vi "Serial_Read (2).vi"() -> ()   [LabVIEW 2010]
uses:
  <vilib>/Instr/_visa.llb/VISA Configure Serial Port (Instr).vi
  <vilib>/Analysis/NI_AALPro.lvlib
panel:
  in  "Tab Control":T1(tab)
  in  "Serial Input":refnum<visa-resource-name>="COM4"
  in  "data bits":u16=8 min=5 max=8 step=1
  in  "parity":u16(ring) items=["None", "Odd", "Even", "Mark", "Space"]
  in  "stop bits":u16(ring)=10 items=["1.0"=10, "1.5"=15, "2.0"=20]
  in  "flow control":u16(ring) items=["None"=0, "XON/XOFF"=1, "RTS/CTS"=2, "DTR/DSR"=4]
  in  "delay before read (ms)":u32=500
  in  "byte count":u32=500
  out "Incoming Serial String":string
  out "Time":string
  out "Date":string
  in  "stop":bool
  out "return count":u32
  in  "baud rate (9600)":u32=9600
  out "N2O is FLAT":bool
  out "Rolling CO Slope Fit":cluster{i32[], "Best Linear Fit":dbl[]}[](graph)
  out "CO":dbl(graph)=0.310407
  out "N2O":dbl(graph)
  out "H2O":dbl(graph)
  out "CO PPM":string
  out "N2O PPM":string
  out "H2O PPM":string
  out "CO DRY":dbl(graph)
  out "CO DRY":string
  out "N2O DRY 2":string
  out "N2O DRY":dbl(graph)
  in  "Average Points":i32
  out "slope":dbl
  out "Rolling N2O Slope Fit 2":cluster{i32[], "Best Linear Fit":dbl[]}[](graph)
  out "slope 2":dbl
  in  "N2O Low Limit":dbl
  in  "CO High Limit":dbl
  out "CO is FLAT":bool
  in  "CO Low Limit":dbl
  in  "N2O High Limit":dbl
  out "CELL TEMP":string
  out "CELL TEMPERATURE":dbl(graph)
  out "AMBIENT TEMPERATURE":dbl(graph)
  out "AMBIENT TEMP":string
  out "AIN5":dbl(graph)
  out "SUPERCOOL TEMP":string
  out "LINE LOCK":dbl(graph)
  out "LINELOCK - LASER CONTROL VOLTAGE":string
  out "PRESSURE":dbl(graph)
  out "PRESSURE 2":string
  out "SuperCool Temperature":dbl
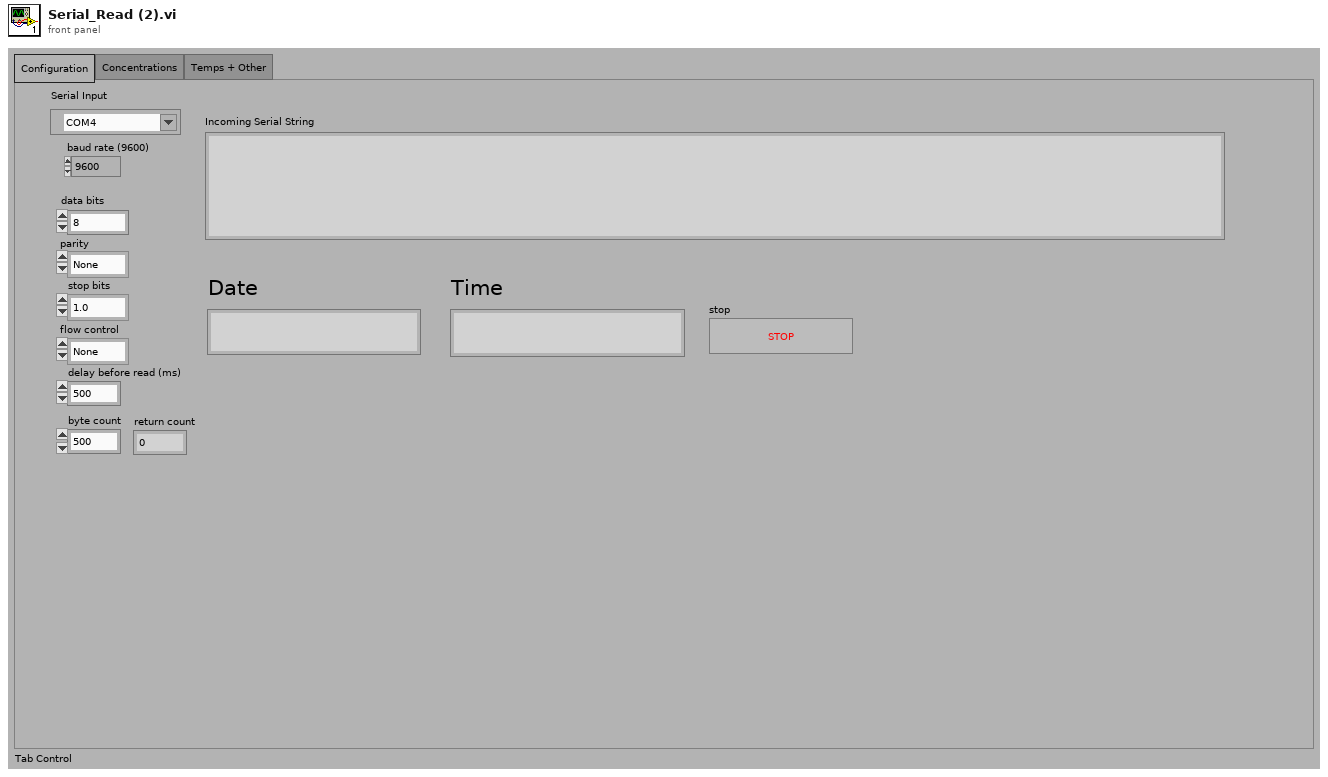
[diagram p1: front panel]
types:
  T1 = enum32{"Configuration", "Concentrations", "Temps + Other"}
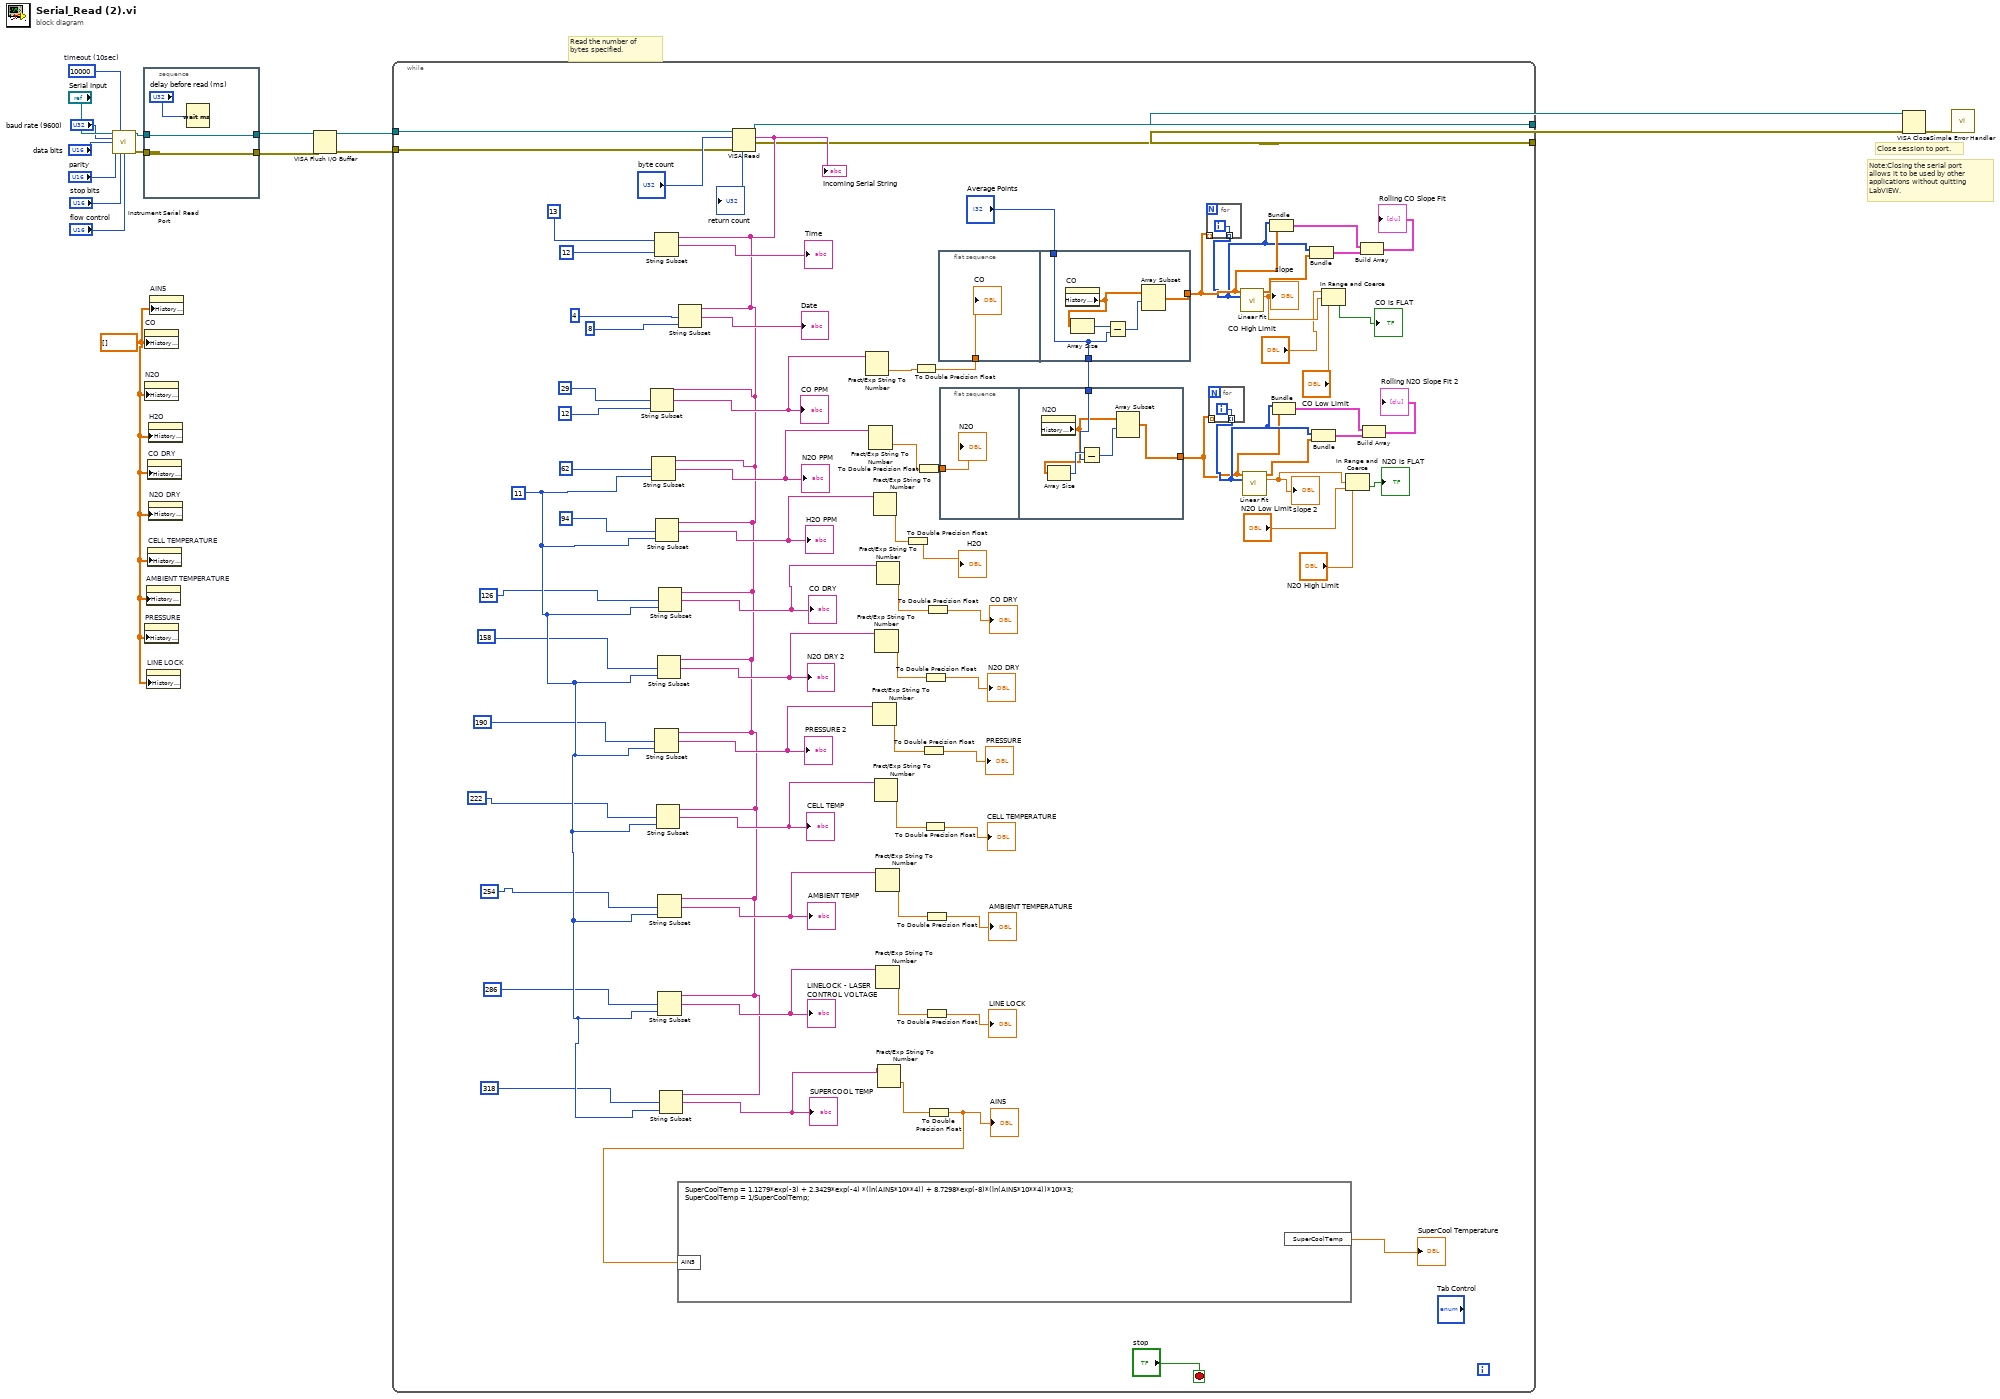
[diagram p0: block diagram]
diagram:
  w2 = dbl[] [] ("History Data")
  w14 = u32 10000  # timeout (10sec)
  # "Read the number of bytes specified."
  # "Note:Closing the serial port allows it to be used by other applications without quitting LabVIEW."
  # "Close session to port."
  n1 = call-poly "Instrument Serial Read Port"("VISA resource name"="Serial Input", "timeout (10sec)"=w14, "baud rate (9600)"="baud rate (9600)", "data bits (8)"="data bits", "parity (0:none)"="parity", "stop bits (10: 1 bit)"="stop bits", "flow control (0:none)"="flow control") -> ("VISA resource name out"=w9:refnum<visa-resource-name>, "error out"=w10:errorcluster)  [unwired: 2 in, 5 out]
  n2 = stacked-sequence {
    tunnel: w10 -> [w20]
    tunnel: [w20] -> w3
    tunnel: w9 -> [w19]
    tunnel: [w19] -> w4
    frame #0 {
      n3 = Wait (ms)(milliseconds to wait="delay before read (ms)") -> ()  [unwired: 1 out]
    }
  }
  n4 = property on="CO" class="WFChart (strict)"("History Data"=w2) -> ()  [unwired: 2 in, 2 out]
  n5 = property on="N2O" class="WFChart (strict)"("History Data"=w2) -> ()  [unwired: 2 in, 2 out]
  n6 = property on="PRESSURE" class="WFChart (strict)"("History Data"=w2) -> ()  [unwired: 2 in, 2 out]
  n7 = property on="AMBIENT TEMPERATURE" class="WFChart (strict)"("History Data"=w2) -> ()  [unwired: 2 in, 2 out]
  n8 = property on="LINE LOCK" class="WFChart (strict)"("History Data"=w2) -> ()  [unwired: 2 in, 2 out]
  n9 = property on="CO DRY" class="WFChart (strict)"("History Data"=w2) -> ()  [unwired: 2 in, 2 out]
  n10 = property on="CELL TEMPERATURE" class="WFChart (strict)"("History Data"=w2) -> ()  [unwired: 2 in, 2 out]
  n11 = property on="H2O" class="WFChart (strict)"("History Data"=w2) -> ()  [unwired: 2 in, 2 out]
  n12 = property on="N2O DRY" class="WFChart (strict)"("History Data"=w2) -> ()  [unwired: 2 in, 2 out]
  n13 = property on="AIN5" class="WFChart (strict)"("History Data"=w2) -> ()  [unwired: 2 in, 2 out]
  n14 = VISA Flush I/O Buffer(VISA resource name=w4, error in (no error)=w3) -> (VISA resource name out=w6:refnum<visa-resource-name>, error out=w5:errorcluster)  [unwired: 1 in]
  n15 = while {
    tunnel: w6 -> [w68]
    tunnel: w5 -> [w69]
    tunnel: [w92] -> w8
    tunnel: [w46] -> w7
    stop <- "stop" stop-if-true
    w58 = 11 ("offset (0)")
    n16 = VISA Read(VISA resource name=w68, byte count="byte count", error in (no error)=w69) -> (VISA resource name out=w92:refnum<visa-resource-name>, read buffer=w59:string, return count=→"return count":u32, error out=w46:errorcluster)
    "Incoming Serial String" <- w59
    n17 = String Subset(string=w59, offset (0)=29, length (rest)=12 ("length (rest)")) -> (substring=w86:string)
    "CO PPM" <- w86
    n18 = String Subset(string=w59, offset (0)=62, length (rest)=w58) -> (substring=w85:string)
    "N2O PPM" <- w85
    n19 = String Subset(string=w59, offset (0)=13, length (rest)=12 ("length (rest)")) -> (substring=→"Time":string)
    n20 = String Subset(string=w59, offset (0)=190, length (rest)=w58) -> (substring=w71:string)
    "PRESSURE 2" <- w71
    n21 = String Subset(string=w59, offset (0)=94, length (rest)=w58) -> (substring=w84:string)
    "H2O PPM" <- w84
    n22 = String Subset(string=w59, offset (0)=222, length (rest)=w58) -> (substring=w70:string)
    "CELL TEMP" <- w70
    n23 = String Subset(string=w59, offset (0)=158, length (rest)=w58) -> (substring=w72:string)
    "N2O DRY 2" <- w72
    n24 = String Subset(string=w59, offset (0)=254, length (rest)=w58) -> (substring=w62:string)
    "AMBIENT TEMP" <- w62
    n25 = String Subset(string=w59, offset (0)=286, length (rest)=w58) -> (substring=w61:string)
    "LINELOCK - LASER CONTROL VOLTAGE" <- w61
    n26 = String Subset(string=w59, offset (0)=126, length (rest)=w58) -> (substring=w73:string)
    "CO DRY" <- w73
    n27 = String Subset(string=w59, offset (0)=318, length (rest)=w58) -> (substring=w60:string)
    "SUPERCOOL TEMP" <- w60
    n28 = String Subset(string=w59, offset (0)=4, length (rest)=8 ("length (rest)")) -> (substring=→"Date":string)
    n29 = Fract/Exp String To Number(string=w86) -> (number=w83:dbl)  [unwired: 3 in, 1 out]
    n30 = Fract/Exp String To Number(string=w85) -> (number=w38:dbl)  [unwired: 3 in, 1 out]
    n31 = Fract/Exp String To Number(string=w71) -> (number=w76:dbl)  [unwired: 3 in, 1 out]
    n32 = Fract/Exp String To Number(string=w84) -> (number=w82:dbl)  [unwired: 3 in, 1 out]
    n33 = Fract/Exp String To Number(string=w70) -> (number=w74:dbl)  [unwired: 3 in, 1 out]
    n34 = Fract/Exp String To Number(string=w72) -> (number=w78:dbl)  [unwired: 3 in, 1 out]
    n35 = Fract/Exp String To Number(string=w62) -> (number=w66:dbl)  [unwired: 3 in, 1 out]
    n36 = Fract/Exp String To Number(string=w61) -> (number=w64:dbl)  [unwired: 3 in, 1 out]
    n37 = Fract/Exp String To Number(string=w73) -> (number=w80:dbl)  [unwired: 3 in, 1 out]
    n38 = Fract/Exp String To Number(string=w60) -> (number=w63:dbl)  [unwired: 3 in, 1 out]
    n39 = To Double Precision Float(number=w82) -> (double precision float=→"H2O":dbl)
    n40 = To Double Precision Float(number=w83) -> (double precision float=w45:dbl)
    n41 = To Double Precision Float(number=w38) -> (double precision float=w37:dbl)
    n42 = To Double Precision Float(number=w76) -> (double precision float=→"PRESSURE":dbl)
    n43 = To Double Precision Float(number=w74) -> (double precision float=→"CELL TEMPERATURE":dbl)
    n44 = To Double Precision Float(number=w78) -> (double precision float=→"N2O DRY":dbl)
    n45 = To Double Precision Float(number=w66) -> (double precision float=→"AMBIENT TEMPERATURE":dbl)
    n46 = To Double Precision Float(number=w64) -> (double precision float=→"LINE LOCK":dbl)
    n47 = To Double Precision Float(number=w80) -> (double precision float=→"CO DRY":dbl)
    n48 = To Double Precision Float(number=w63) -> (double precision float=w49:dbl)
    "AIN5" <- w49
    n49 = formula code="SuperCoolTemp = 1.1279*exp(-3) + 2.3429*exp(-4) *(ln(AIN5*10**4)) + 8.7298*exp(-8)*(ln(AIN5*10**4))*10**3;\nSuperCoolTemp = 1/SuperCoolTemp;"("AIN5"=w49) -> ("SuperCoolTemp"=→"SuperCool Temperature":dbl)
    n50 = flat-sequence {
      tunnel: w45 -> [w108]
      tunnel: [w110] -> w44
      tunnel: "Average Points" -> [w109]
      tunnel: [w109] -> w35
      frame #0 {
        "CO" <- w108
      }
      frame #1 {
        n51 = property on="CO" class="WFChart (strict)"() -> ("History Data"=w111:dbl[])  [unwired: 2 in, 2 out]
        n52 = Array Size(array=w111) -> (size(s)=w112:i32)
        n53 = Subtract(x=w112, y=w109) -> (x-y=w113:i32)
        n54 = Array Subset(array=w111, index=w113) -> (w110:dbl[])  [unwired: 1 in]
      }
    }
    n55 = flat-sequence {
      tunnel: w37 -> [w101]
      tunnel: w35 -> [w104]
      tunnel: [w102] -> w29
      frame #0 {
        "N2O" <- w101
      }
      frame #1 {
        n56 = property on="N2O" class="WFChart (strict)"() -> ("History Data"=w103:dbl[])  [unwired: 2 in, 2 out]
        n57 = Array Size(array=w103) -> (size(s)=w105:i32)
        n58 = Subtract(x=w105, y=w104) -> (x-y=w106:i32)
        n59 = Array Subset(array=w103, index=w106) -> (w102:dbl[])  [unwired: 1 in]
      }
    }
    n60 = for {
      tunnel: [w107] -> w43 mode=indexing
      tunnel: w44 -> [_] mode=indexing
      i -> [w107]
    }
    n61 = for {
      tunnel: [w100] -> w34 mode=indexing
      tunnel: w29 -> [_] mode=indexing
      i -> [w100]
    }
    n62 = call <vilib>:"Linear Fit.vi"("Y"=w44, "X"=w43) -> ("Best Linear Fit"=w42:dbl[], "slope"=w28:dbl)  [unwired: 9 in, 3 out]
    "slope" <- w28
    n63 = call <vilib>:"Linear Fit.vi"("Y"=w29, "X"=w34) -> ("Best Linear Fit"=w33:dbl[], "slope"=w23:dbl)  [unwired: 9 in, 3 out]
    "slope 2" <- w23
    n64 = Bundle(w43, w44) -> (w41:cluster{i32[], dbl[]})  [unwired: 1 in]
    n65 = Bundle(w34, w29) -> (w32:cluster{i32[], dbl[]})  [unwired: 1 in]
    n66 = Bundle(w43, "Best Linear Fit"=w42) -> (w40:cluster{i32[], "Best Linear Fit":dbl[]})  [unwired: 1 in]
    n67 = Bundle(w34, "Best Linear Fit"=w33) -> (w31:cluster{i32[], "Best Linear Fit":dbl[]})  [unwired: 1 in]
    n68 = In Range and Coerce(upper limit="CO High Limit", x=w28, lower limit="CO Low Limit") -> (In Range?=→"CO is FLAT":bool)  [unwired: 1 out]
    n69 = In Range and Coerce(upper limit="N2O High Limit", x=w23, lower limit="N2O Low Limit") -> (In Range?=→"N2O is FLAT":bool)  [unwired: 1 out]
    n70 = Build Array(w41, w40) -> (→"Rolling CO Slope Fit":cluster{i32[], "Best Linear Fit":dbl[]}[])
    n71 = Build Array(w32, w31) -> (→"Rolling N2O Slope Fit 2":cluster{i32[], "Best Linear Fit":dbl[]}[])
  }
  n72 = VISA Close(VISA resource name=w8, error in (no error)=w7) -> (error out=w16:errorcluster)
  n73 = call <vilib>:"Simple Error Handler.vi"("error in (no error)"=w16) -> ()  [unwired: 1 in, 8 out]
